vi "PUT Number of Sweeps.vi"(0 "Number of Sweeps":dbl) -> ()   [LabVIEW 2013]
uses:
  Action.ctl
  Power Peak Calibration Input FGV Selector.ctl
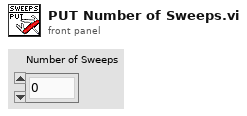
[diagram p1: front panel]
types:
  T1 = typedef "Power Peak Calibration Input FGV Selector.ctl" = enum16{"Samples/Sweep", "Num Sweeps", "Sample Rate"}
  T2 = typedef "Action.ctl" = enum16{"GET", "PUT", "DELETE"}
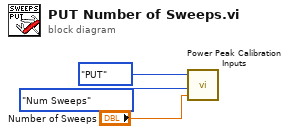
[diagram p0: block diagram]
diagram:
  n1 = call "Power Peak Calibration Inputs.vi"("Input"="Number of Sweeps", "Calibration Input FGV Selector"=Power_Peak_Calibration_Input_FGV_Selector."Num Sweeps", "Verb"=Action."PUT") -> ()  [unwired: 1 out]
